vi "GetTestPcNames.vi"(8 "error in (no error)":errorcluster) -> (0 "error out":errorcluster, 1 "IP":string, 2 "Basic Name":string, 3 "Computer Full Name":string, 4 "Production test pc?":bool)   [LabVIEW 2013]
uses:
  Test Globals/Global 1.vi
panel:
  out "Test pc list":string
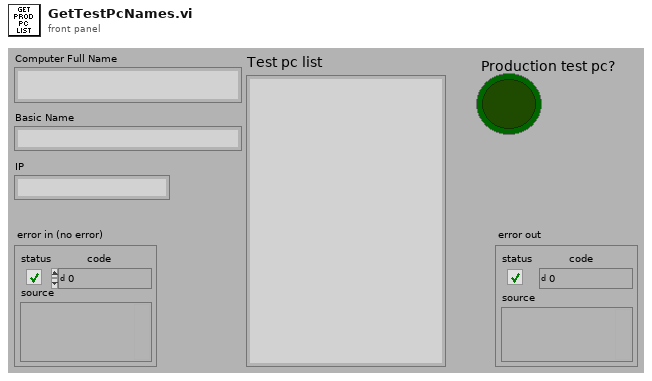
[diagram p1: front panel]
types:
  T1 = cluster{"Test folder":string, "Top level":string, "Main":string, "Test report":string, "Work order qty":string, "Work order meid":string, "Work order imei":string, "Master meid imei list":string, "Master test data":string, "ZPL label info":string, "Pictures":string, "Setup info":string, "Work order":string, "Tests folder":string, "Tests steps folder":string, "Config folder":string, "Verizon Upload file":string, "Job data file":string, "Station globals":string, "Post test info":string}
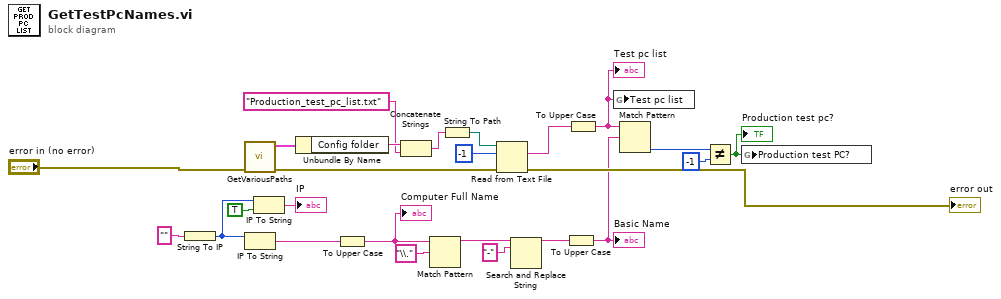
[diagram p0: block diagram]
diagram:
  n1 = String To IP(1:"" ("name")) -> (0:w23:u32)
  n2 = call "GetVariousPaths.vi"("error in (no error)"="error in (no error)") -> ("error out"=w14:errorcluster, "Built Paths"=w16:T1)  [unwired: 9 in]
  n3 = IP To String(2:w23) -> (0:w3:string)  [unwired: 1 in]
  n4 = IP To String(1:TRUE ("dot notation? (F)"), 2:w23) -> (0:→"IP":string)
  n5 = Unbundle By Name(w16) -> ("Config folder"=w15:string)
  n6 = To Upper Case(1:w3) -> (0:w2:string)
  "Computer Full Name" <- w2
  n7 = Concatenate Strings(w15, "Production_test_pc_list.txt" ("string")) -> (w18:string)
  n8 = Match Pattern(string=w2, regular expression="\\.") -> (before substring=w20:string)  [unwired: 1 in, 3 out]
  n9 = String To Path(string=w18) -> (path=w9:path)
  n10 = Read from Text File(file (use dialog)=w9, count=-1, error in=w14) -> (text=w7:string, error out=→"error out":errorcluster)  [unwired: 1 in, 2 out]
  n11 = Search and Replace String(input string=w20, search string="-") -> (result string=w5:string)  [unwired: 6 in, 3 out]
  n12 = To Upper Case(1:w5) -> (0:w1:string)
  "Basic Name" <- w1
  n13 = To Upper Case(1:w7) -> (0:w6:string)
  "Test pc list" <- w6
  n14 = global write "Global 1.vi" "Test pc list"(w6) -> ()
  n15 = Match Pattern(string=w6, regular expression=w1) -> (offset past match=w12:i32)  [unwired: 1 in, 3 out]
  n16 = Not Equal?(x=w12, y=-1) -> (x != y?=w8:bool)
  "Production test pc?" <- w8
  n17 = global write "Global 1.vi" "Production test PC?"(w8) -> ()
